vi "Day 04 Part 2.vi"(11 "Input":string) -> (3 "Output":u32)   [LabVIEW 2021]
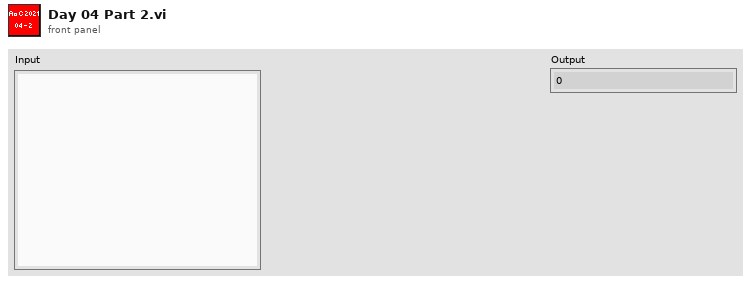
[diagram p1: front panel]
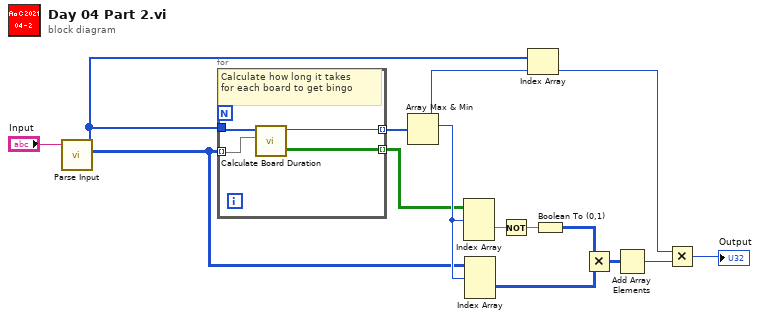
[diagram p0: block diagram]
diagram:
  n1 = call "Parse Input.vi"("Input"="Input") -> ("Boards"=w2:i32[][][], "Draw"=w8:i32[])  [unwired: 9 in]
  n2 = for {
    tunnel: w2 -> [w18] mode=indexing
    tunnel: w8 -> [w19]
    tunnel: [w17] -> w15 mode=indexing
    tunnel: [w16] -> w1 mode=indexing
    # "Calculate how long it takes\nfor each board to get bingo"
    n3 = call "Calculate Board Duration.vi"("Board"=w18, "Draw"=w19) -> ("Marked"=w16:bool[][], "Duration"=w17:i32)  [unwired: 6 in, 2 out]
  }
  n4 = Array Max & Min(array=w15) -> (max value=w4:i32, max index (indices)=w5:i32)  [unwired: 2 out]
  n5 = Index Array(array=w1, index (dim 0)=w5) -> (element=w3:bool[][])  [unwired: 2 in]
  n6 = Index Array(array=w2, index (dim 0)=w5) -> (element=w12:i32[][])  [unwired: 2 in]
  n7 = Not(x=w3) -> (.not. x?=w13:bool[][])
  n8 = Index Array(array=w8, index=w4) -> (element=w14:i32)
  n9 = Boolean To (0,1)(Boolean=w13) -> (0, 1=w11:i16[][])
  n10 = Multiply(x=w11, y=w12) -> (x*y=w10:i32[][])
  n11 = Add Array Elements(numeric array=w10) -> (sum=w9:i32)
  n12 = Multiply(x=w14, y=w9) -> (x*y=→"Output":i32)
